vi "FpgaInit.vi"(8 "error in (no error)":errorcluster, 11 "AODAcq in":refnum<class "AODAcq.lvclass">) -> (0 "error out":errorcluster, 3 "AODAcq out":refnum<class "AODAcq.lvclass">)   [LabVIEW 2014, in "AODAcq.lvclass"]
uses:
  AODAcq.lvclass
  FPGA_Control/AODRef.ctl
  <vilib>/rvi/interface/nirviOpenFPGA/nirviOpenFPGA.xnode
  <vilib>/rvi/interface/nirviMethod/nirviMethod.xnode
  <vilib>/LabVIEW Targets/FPGA/RIO/nirio_PxiTriggers.ctl
  <vilib>/rvi/interface/nirviReadWriteControl/nirviReadWriteControl.xnode
  <vilib>/userdefined/High Color/nirio_resource_hc.ctl
  <vilib>/rvi/errors/niLvFpgaMergeErrorWithErrorCode.vi
  <vilib>/FPGA/interface/niFpgaViExecutionMode.ctl
  <vilib>/Utility/error.llb/Error Cluster From Error Code.vi
  <vilib>/rvi/errors/niLvFpgaAdjustHostInterfaceError.vi
  NiFpgaLv.dll
  <vilib>/FPGAPlugInAG/PXIe-7965R/niLvFpga_ConfigureFifo_PXIe-7965R.vi
  <vilib>/FPGAPlugInAG/PXIe-7965R/niLvFpga_StartFifo_PXIe-7965R.vi
  <vilib>/FPGAPlugInAG/PXIe-7965R/niLvFpga_Reset_PXIe-7965R.vi
  <vilib>/FPGAPlugInAG/PXIe-7965R/niLvFpga_Run_PXIe-7965R.vi
  FPGA Bitfiles/AodScanner_FPGATarget_AODControl(FPGA)_TyJc9yYmyGA.lvbitx
  <vilib>/FPGAPlugInAG/PXIe-7965R/niLvFpga_Open_PXIe-7965R.vi
  <vilib>/LabVIEW Targets/FPGA/RIO/nirioReserveTrigger.vi
  <vilib>/LabVIEW Targets/FPGA/FlexRIO/CustomFPGAMethods/79XXR_Method_IOModuleStatusImpl.vi
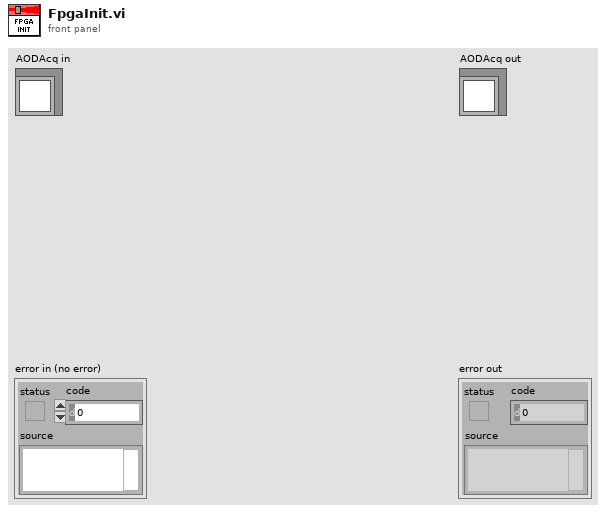
[diagram p1: front panel]
types:
  T1 = typedef "nirio_resource_hc.ctl" = tag
  T2 = typedef "AODRef.ctl" = refnum<k20>
  T3 = typedef "niFpgaViExecutionMode.ctl" = enum16{"FPGA Target", "Simulation (Simulated I/O)", "Simulation (Real I/O)", "Third-Party Simulation"}
  T4 = typedef "nirio_PxiTriggers.ctl" = u16
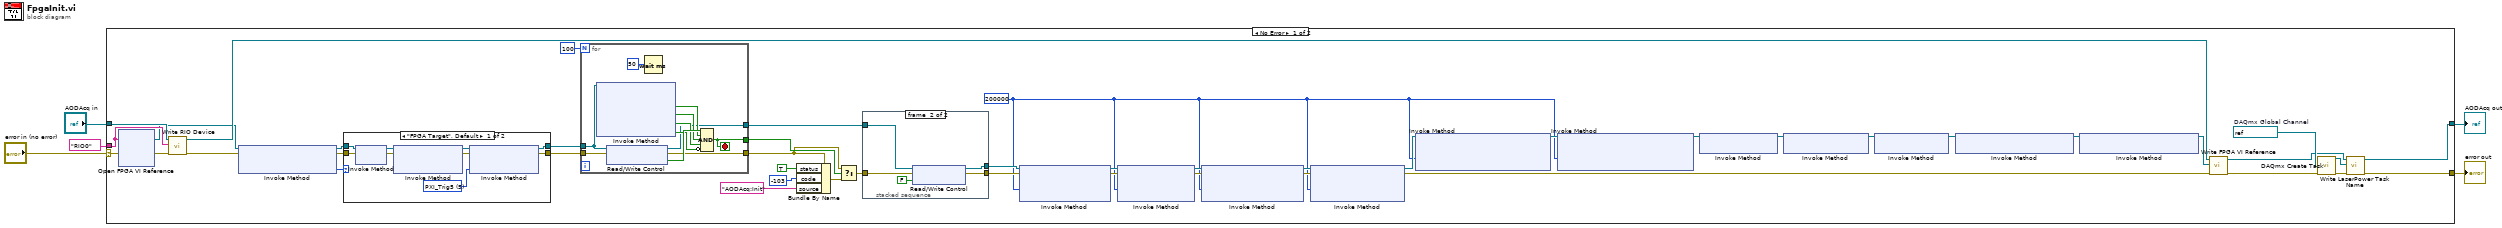
[diagram p0: block diagram]
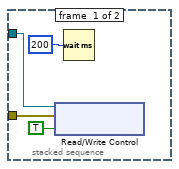
[diagram p2: hidden frame]
diagram:
  n1 = case shown="No Error" "error in (no error)" {
    selector: "error in (no error)" -> [w49 w84]
    tunnel: [w40 w84] -> w3
    tunnel: [w41 w83] -> w4
    tunnel: "AODAcq in" -> [w39 w83]
    tunnel: T1 "RIO0" ("RIO Device") -> [w37 _]
    frame No Error {
      w46 = refnum<k21> "AOD Gain"  # DAQmx Global Channel
      w6 = u32 200000 ("Depth")
      n2 = xnode "Open FPGA VI Reference"("error in"=w49, "resource name"=w37) -> ("FPGA VI Reference Out"=w13:T2, "error out"=w36:errorcluster)
      n3 = call-dynamic "Write RIO Device.vi"("error in (no error)"=w36, "RIO Device"=w37, "AODAcq in"=w39) -> ("error out"=w35:errorcluster, "AODAcq out"=w38:refnum<class "AODAcq.lvclass">)  [unwired: 7 in]
      n4 = xnode "Invoke Method"("FPGA VI Reference In"=w13, "error in"=w35) -> ("FPGA VI Reference Out"=w51:T2, "error out"=w48:errorcluster, "FPGA VI Execution Mode"=w50:T3)
      n5 = case shown="\"FPGA Target\", Default" w50 {
        tunnel: [w76 w82] -> w34
        tunnel: w51 -> [w80 w82]
        tunnel: w48 -> [w75 w81]
        tunnel: [w72 w81] -> w33
        frame "FPGA Target", Default {
          w78 = T4 5 items=["PXI_Trig0", "PXI_Trig1", "PXI_Trig2", "PXI_Trig3", "PXI_Trig4", "PXI_Trig5", "PXI_Trig6", "PXI_Trig7"] ("Trigger")
          n6 = xnode "Invoke Method"("FPGA VI Reference In"=w80, "error in"=w75) -> ("FPGA VI Reference Out"=w79:T2, "error out"=w74:errorcluster)
          n7 = xnode "Invoke Method"("FPGA VI Reference In"=w79, "error in"=w74) -> ("FPGA VI Reference Out"=w77:T2, "error out"=w73:errorcluster)  [unwired: 1 in]
          n8 = xnode "Invoke Method"("FPGA VI Reference In"=w77, "error in"=w73, "Trigger"=w78) -> ("FPGA VI Reference Out"=w76:T2, "error out"=w72:errorcluster)
        }
        frame "Simulation (Simulated I/O)" {
        }
      }
      n9 = for {
        N: 100 -> [_]
        tunnel: w34 -> [w61]
        tunnel: w33 -> [w62]
        tunnel: [w53] -> w32
        tunnel: [w55] -> w30
        tunnel: [w52] -> w25
        stop <- w53 stop-if-true
        n10 = xnode "Invoke Method"("FPGA VI Reference In"=w61) -> ("IO Module Present?"=w59:bool, "Power Enabled?"=w58:bool, "IO Enabled?"=w57:bool, "IO Module Mismatch?"=w56:bool)  [unwired: 1 in, 2 out]
        n11 = xnode "Read/Write Control"("FPGA VI Reference In"=w61, "error in"=w62) -> ("FPGA VI Reference Out"=w52:T2, "error out"=w55:errorcluster, "Status.Initialized"=w60:bool)
        n12 = Wait (ms)(milliseconds to wait=u32 50) -> ()  [unwired: 1 out]
        n13 = Compound Arithmetic op=AND(w60, w59, w58, w57, invert w56) -> (w53:bool)
      }
      n14 = Bundle By Name(cluster=w30, "status"=TRUE, "code"=-103, "source"="AODAcq:Init") -> (w29:errorcluster)
      n15 = Select(t=w30, s=w32, f=w29) -> (s? t:f=w24:errorcluster)
      n16 = stacked-sequence {
        tunnel: w25 -> [w66 w71]
        tunnel: w24 -> [w65 w70]
        tunnel: [_ w68] -> w15
        tunnel: [_ w67] -> w14
        frame #0 {
          n17 = xnode "Read/Write Control"("FPGA VI Reference In"=w66, "error in"=w65, "Control.Reset"=TRUE) -> ()  [unwired: 2 out]
          n18 = Wait (ms)(milliseconds to wait=u32 200) -> ()  [unwired: 1 out]
        }
        frame #1 {
          n19 = xnode "Read/Write Control"("FPGA VI Reference In"=w71, "error in"=w70, "Control.Reset"=FALSE) -> ("FPGA VI Reference Out"=w68:T2, "error out"=w67:errorcluster)
        }
      }
      n20 = xnode "Invoke Method"("FPGA VI Reference In"=w15, "error in"=w14, "Requested Depth"=w6) -> ("FPGA VI Reference Out"=w18:T2, "error out"=w47:errorcluster)  [unwired: 1 out]
      n21 = xnode "Invoke Method"("FPGA VI Reference In"=w18, "error in"=w47, "Requested Depth"=w6) -> ("FPGA VI Reference Out"=w23:T2, "error out"=w22:errorcluster)  [unwired: 1 out]
      n22 = xnode "Invoke Method"("FPGA VI Reference In"=w23, "error in"=w22, "Requested Depth"=w6) -> ("FPGA VI Reference Out"=w21:T2, "error out"=w20:errorcluster)  [unwired: 1 out]
      n23 = xnode "Invoke Method"("FPGA VI Reference In"=w21, "error in"=w20, "Requested Depth"=w6) -> ("FPGA VI Reference Out"=w11:T2, "error out"=w19:errorcluster)  [unwired: 1 out]
      n24 = xnode "Invoke Method"("FPGA VI Reference In"=w11, "Requested Depth"=w6) -> ("FPGA VI Reference Out"=w12:T2)  [unwired: 1 in, 2 out]
      n25 = xnode "Invoke Method"("FPGA VI Reference In"=w12, "Requested Depth"=w6) -> ("FPGA VI Reference Out"=w10:T2)  [unwired: 1 in, 2 out]
      n26 = xnode "Invoke Method"("FPGA VI Reference In"=w10) -> ("FPGA VI Reference Out"=w17:T2)  [unwired: 1 in, 1 out]
      n27 = xnode "Invoke Method"("FPGA VI Reference In"=w17) -> ("FPGA VI Reference Out"=w16:T2)  [unwired: 1 in, 1 out]
      n28 = xnode "Invoke Method"("FPGA VI Reference In"=w16) -> ("FPGA VI Reference Out"=w9:T2)  [unwired: 1 in, 1 out]
      n29 = xnode "Invoke Method"("FPGA VI Reference In"=w9) -> ("FPGA VI Reference Out"=w8:T2)  [unwired: 1 in, 1 out]
      n30 = xnode "Invoke Method"("FPGA VI Reference In"=w8) -> ("FPGA VI Reference Out"=w7:T2)  [unwired: 1 in, 1 out]
      n31 = call-dynamic "Write FPGA VI Reference.vi"("error in (no error)"=w19, "AOD FPGA"=w7, "AODAcq in"=w38) -> ("error out"=w45:errorcluster, "AODAcq out"=w42:refnum<class "AODAcq.lvclass">)  [unwired: 7 in]
      n32 = call <vilib>:"DAQmx Create Task.vi"("global virtual channels"=w46, "error in"=w45) -> ("task out"=w43:refnum<k21>, "error out"=w44:errorcluster)  [unwired: 3 in, 9 out]
      n33 = call-dynamic "Write LaserPower Task Name.vi"("error in (no error)"=w44, "LaserPower Task Name"=w43, "AODAcq in"=w42) -> ("error out"=w40:errorcluster, "AODAcq out"=w41:refnum<class "AODAcq.lvclass">)  [unwired: 7 in]
    }
    frame Error {
    }
  }
  "error out" <- w3
  "AODAcq out" <- w4
